vi "盘显示.vi"() -> ()   [LabVIEW 2016]
uses:
  <userlib>/_OpenG.lib/numeric/numeric.llb/Random Number Within Range - I32__ogtk.vi
panel:
  out "二维图片":picture
  in  "起点":cluster{"x":i32, "y":i32}={"x"=20, "y"=20}
  in  "块大小":cluster{"x":dbl, "y":dbl}={"x"=50.0, "y"=25.0}
  in  "行列数":cluster{"x":i32, "y":i32}={"x"=10, "y"=10}
  in  "间距":cluster{"x":i32, "y":i32}={"x"=100, "y"=50}
  out "选中的ID":i32=24
  in  "画图":bool
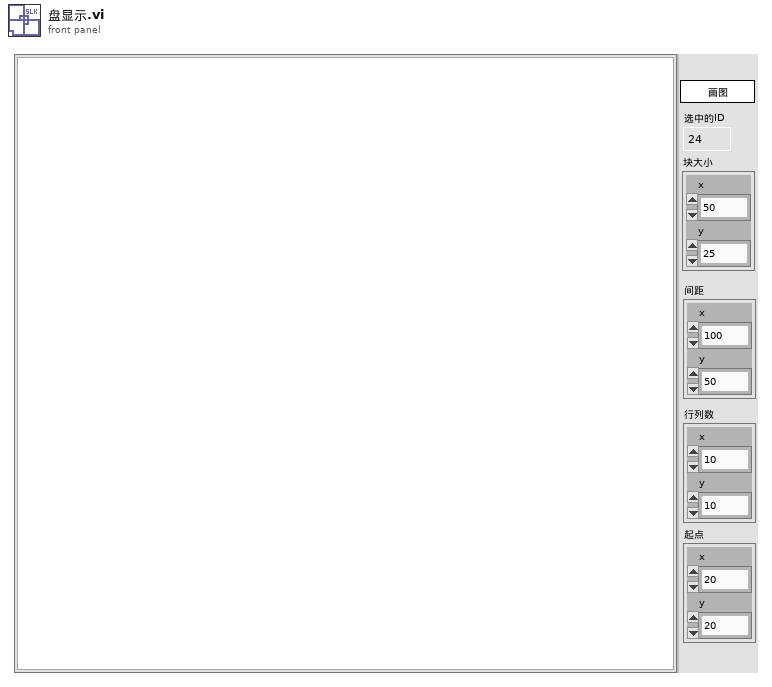
[diagram p1: front panel]
types:
  T1 = cluster{"rect":cluster{"left":i16, "top":i16, "right":i16, "bottom":i16}, "颜色":u32, "ID":string}
  T2 = cluster{"left":i16, "top":i16, "right":i16, "bottom":i16}
  T3 = typedef "LVPoint32TypeDef.ctl" = cluster{"Horizontal":i32, "Vertical":i32}
  T4 = cluster{"rect":cluster{"left":i16, "top":i16, "right":i16, "bottom":i16}, "颜色":u32, "ID":string}[]
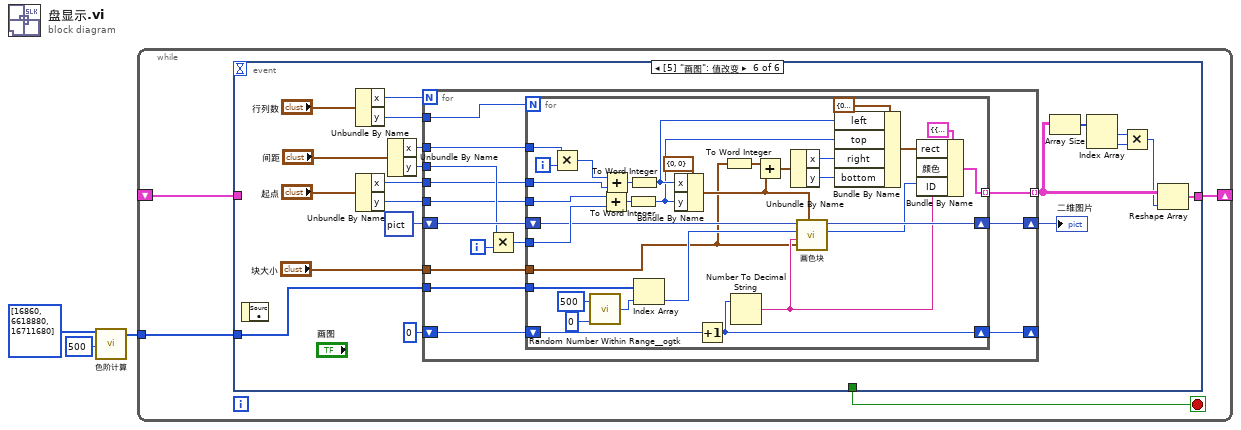
[diagram p0: block diagram]
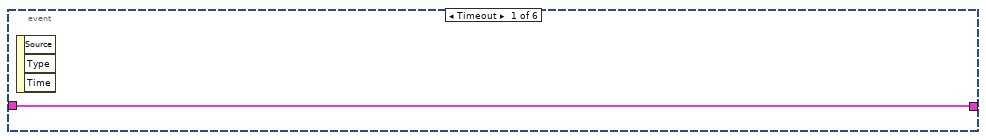
[diagram p2: hidden frame]
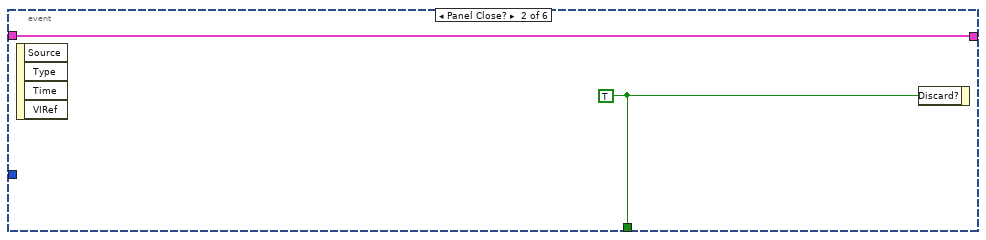
[diagram p3: hidden frame]
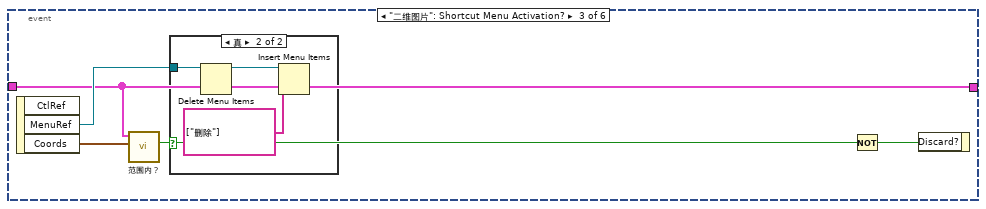
[diagram p4: hidden frame]
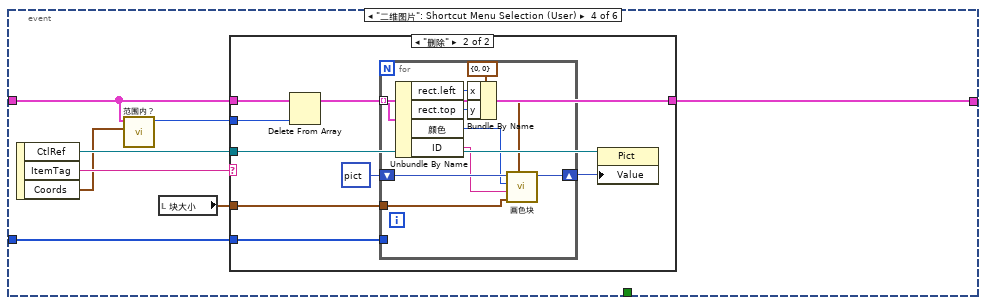
[diagram p6: hidden frame]
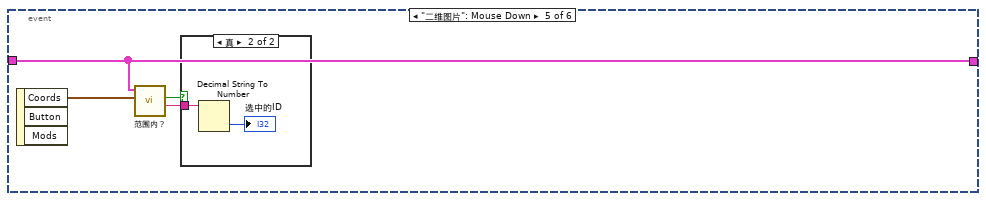
[diagram p8: hidden frame]
diagram:
  n1 = call "色阶计算.vi"("多个颜色盒"=u32[] [16860, 6618880, 16711680], "阶数"=500) -> ("色阶"=w1:u32[])  [unwired: 17 in]
  n2 = while {
    shift-right: [w6] -> _
    shift-left: _ -> [w4]
    tunnel: w1 -> [w5]
    stop <- w7 stop-if-true
    n3 = event shown="[5] \"画图\": 值改变" {
      selector: _ -> [_ _ _ _ _ _]
      dyn-events: _ -> [_ _ _ _ _ _]
      timeout: _ -> [_ _ _ _ _ _]
      tunnel: [_ w10 _ _ _ _] -> w7
      tunnel: [w8 w9 w11 w21 w46 w68] -> w6
      tunnel: w5 -> [_ _ _ w22 _ w60]
      tunnel: w4 -> [w8 w9 w11 w19 w46 _]
      event Timeout {
        n4 = event-data() -> ()  [unwired: 1 in, 3 out]
      }
      event Panel Close? {
        w10 = TRUE
        n5 = event-data() -> ()  [unwired: 1 in, 4 out]
        n6 = event-data("Discard?"=w10) -> ()  [unwired: 1 in, 1 out]
      }
      event "二维图片": Shortcut Menu Activation? {
        n7 = event-data() -> ("MenuRef"=w15:refnum<k9>, "Coords"=w13:T3)  [unwired: 1 in, 1 out]
        n8 = call "范围内？.vi"("Coords"=w13, "数组"=w11) -> ("pt in rect"=w12:bool)  [unwired: 7 in, 2 out]
        n9 = case shown="真" w12 {
          tunnel: w15 -> [_ w18]
          frame False {
          }
          frame True {
            n10 = Delete Menu Items(9:w18) -> (3:w17:refnum<k9>)  [unwired: 3 in, 1 out]
            n11 = Insert Menu Items(7:string[] ["删除"] ("项标识符"), 9:w17) -> ()  [unwired: 4 in, 3 out]
          }
        }
        n12 = Not(x=w12) -> (.not. x?=w14:bool)
        n13 = event-data("Discard?"=w14) -> ()  [unwired: 1 in, 1 out]
      }
      event "二维图片": Shortcut Menu Selection (User) {
        n14 = event-data() -> ("CtlRef"=w25:refnum<vi>, "ItemTag"=w26:string, "Coords"=w24:T3)  [unwired: 1 in]
        n15 = call "范围内？.vi"("Coords"=w24, "数组"=w19) -> ("Index"=w23:i32)  [unwired: 7 in, 2 out]
        n16 = local read "块大小"() -> (w20:cluster{"x":dbl, "y":dbl})
        n17 = case shown="\"删除\"" w26 {
          tunnel: w25 -> [_ w34]
          tunnel: w23 -> [_ w32]
          tunnel: [w27 w31] -> w21
          tunnel: w22 -> [_ w30]
          tunnel: w20 -> [_ w29]
          tunnel: w19 -> [w27 w28]
          frame "", Default {
          }
          frame "删除" {
            n18 = Delete From Array(array=w28, index=w32) -> (array with subset deleted=w31:T4)  [unwired: 1 in, 1 out]
            n19 = for {
              shift-right: [w45] -> w35
              shift-left: picture data[5B] ("new picture") -> [w44]
              tunnel: w30 -> [_]
              tunnel: w31 -> [w40] mode=indexing
              tunnel: w29 -> [w41]
              n20 = Unbundle By Name(w40) -> ("rect.left"=w39:i16, "rect.top"=w38:i16, "颜色"=w37:u32, "ID"=w36:string)
              n21 = Bundle By Name(cluster=cluster{"x":i16, "y":i16} {"x"=0, "y"=0} ("top left point(0, 0)"), "x"=w39, "y"=w38) -> (w42:cluster{"x":i16, "y":i16})
              n22 = call "画色块.vi"("位置"=w42, "块大小"=w41, "ID"=w36, "颜色"=w37, "picture in"=w44) -> ("picture out"=w45:picture)  [unwired: 6 in]
            }
            n23 = property class="Pict"(reference=w34, "Value"=w35) -> ()  [unwired: 1 in, 2 out]
          }
        }
      }
      event "二维图片": Mouse Down {
        n24 = event-data() -> ("Coords"=w49:T3)  [unwired: 1 in, 2 out]
        n25 = call "范围内？.vi"("Coords"=w49, "数组"=w46) -> ("ID"=w47:string, "pt in rect"=w48:bool)  [unwired: 7 in, 1 out]
        n26 = case shown="真" w48 {
          tunnel: w47 -> [_ w51]
          frame False {
          }
          frame True {
            n27 = Decimal String To Number(string=w51) -> (number=→"选中的ID":i32)  [unwired: 2 in, 1 out]
          }
        }
      }
      event "画图": Value Change {
        n28 = event-data() -> ()  [unwired: 1 in, 1 out]
        n29 = Unbundle By Name("行列数") -> ("x"=w59:i32, "y"=w58:i32)
        n30 = Unbundle By Name("起点") -> ("x"=w57:i32, "y"=w56:i32)
        n31 = Unbundle By Name("间距") -> ("x"=w61:i32, "y"=w62:i32)
        n32 = for {
          N: w59 -> [_]
          shift-right: [w85] -> w71
          shift-left: picture data[5B] ("new picture") -> [w84]
          tunnel: w58 -> [w83]
          shift-right: [w80] -> _
          shift-left: 0 -> [w79]
          tunnel: w60 -> [w78]
          tunnel: [w77] -> w67 mode=indexing
          tunnel: w62 -> [w76]
          tunnel: w61 -> [w75]
          tunnel: w57 -> [w74]
          tunnel: w56 -> [w73]
          tunnel: "块大小" -> [w72]
          i -> [w82]
          n33 = Multiply(x=w76, y=w82) -> (x*y=w81:i32)
          n34 = for {
            N: w83 -> [_]
            shift-right: [w92] -> w85
            shift-left: w84 -> [w94]
            tunnel: w81 -> [w114]
            shift-right: [w112] -> w80
            shift-left: w79 -> [w111]
            tunnel: w78 -> [w105]
            tunnel: [w95] -> w77 mode=indexing
            tunnel: w75 -> [w101]
            tunnel: w74 -> [w88]
            tunnel: w73 -> [w87]
            tunnel: w72 -> [w86]
            i -> [w113]
            n35 = Multiply(x=w101, y=w113) -> (x*y=w115:i32)
            n36 = call-poly <userlib>:"Random Number Within Range__ogtk.vi"("High"=500, "Low"=0) -> ("Random Number"=w106:i32)  [unwired: 3 in]
            n37 = Add(x=w87, y=w114) -> (x+y=w109:i32)
            n38 = Add(x=w115, y=w88) -> (x+y=w110:i32)
            n39 = To Word Integer(number=w109) -> (16bit integer=w102:i16)
            n40 = To Word Integer(number=w110) -> (16bit integer=w103:i16)
            n41 = Index Array(array=w105, index=w106) -> (element=w91:u32)
            n42 = Bundle By Name(cluster=cluster{"x":i16, "y":i16} {"x"=0, "y"=0} ("top left point(0, 0)"), "x"=w103, "y"=w102) -> (w93:cluster{"x":i16, "y":i16})
            n43 = Increment(x=w111) -> (x+1=w112:i32)
            n44 = To Word Integer(number=w86) -> (16bit integer=w89:cluster{"x":i16, "y":i16})
            n45 = Number To Decimal String(number=w112) -> (decimal integer string=w90:string)  [unwired: 1 in]
            n46 = Add(x=w89, y=w93) -> (x+y=w100:cluster{"x":i16, "y":i16})
            n47 = Unbundle By Name(w100) -> ("x"=w99:i16, "y"=w98:i16)
            n48 = call "画色块.vi"("位置"=w93, "块大小"=w86, "ID"=w90, "颜色"=w91, "picture in"=w94) -> ("picture out"=w92:picture)  [unwired: 6 in]
            n49 = Bundle By Name(cluster=T2 {"left"=0, "top"=0, "right"=0, "bottom"=0} ("rect"), "left"=w103, "top"=w102, "right"=w99, "bottom"=w98) -> (w97:T2)
            n50 = Bundle By Name(cluster=T1 {"rect"={"left"=0, "top"=0, "right"=0, "bottom"=0}, "颜色"=16448250, "ID"=""} ("输出簇"), "rect"=w97, "颜色"=w91, "ID"=w90) -> (w95:T1)
          }
        }
        "二维图片" <- w71
        n51 = Array Size(array=w67) -> (size(s)=w66:i32[])
        n52 = Index Array(array=w66) -> (element #1=w64:i32, element #2=w65:i32)  [unwired: 2 in]
        n53 = Multiply(x=w64, y=w65) -> (x*y=w63:i32)
        n54 = Reshape Array(w67, w63) -> (w68:T4)
      }
    }
  }
